vi "Read Model Ref.vi"(11 "IViewModel In":refnum<class "IViewModel.lvclass">) -> (2 "Model Enqueuer":refnum<class "Message Enqueuer.lvclass">)   [LabVIEW 2015, in "IViewModel.lvlib" / "IViewModel.lvclass"]
doc: "<License>\nCopyright © 2017 Composed Systems, LLC | All rights reserved\nwww.composed.io\n\nAuthor: Ethan Stern <ethan.stern@composed.io>\n\nThis software is provided \"AS IS\" WITHOUT WARRANTIES, either express or implied, AND IS FOR EDUCATIONAL PURPOSES ONLY.\n</License>"
uses:
  IViewModel.lvclass
  <vilib>/ActorFramework/Message Enqueuer/Message Enqueuer.lvclass
  IViewModel.lvclass/IViewModel.ctl
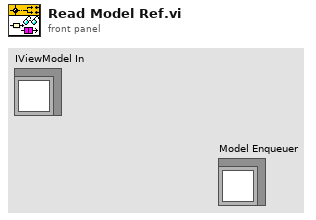
[diagram p1: front panel]
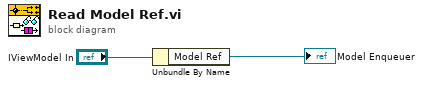
[diagram p0: block diagram]
diagram:
  n1 = Unbundle By Name("IViewModel In") -> ("Model Ref"=→"Model Enqueuer":refnum<class "Message Enqueuer.lvclass">)
